vi "Launch PPMS2 UI.vi"() -> ()   [LabVIEW 2016, in "Instrument.PPMS2 UI.lvclass"]
doc: "This will launch a stan-alone user interface for the PPMS 2 Instrument\n\nJKI State Machine Objects (SMO) 1.0.0.5\nJKI - JKI\nCopyright (c) 2016, JKI"
uses:
  Instrument.PPMS2 UI.lvclass
  C:/Program Files (x86)/National Instruments/LabVIEW 2016/vi.lib/JKI/JKI SMO/SMO/SMO.lvclass
  C:/Program Files (x86)/National Instruments/LabVIEW 2016/vi.lib/JKI/JKI SMO/SMO.UI/SMO.UI.lvclass
  instrument.PPMS2/instrument.PPMS2.lvclass
  C:/Program Files (x86)/National Instruments/LabVIEW 2016/user.lib/LevyLab/Levylab Instruments/SMOs/Instrument/Instrument.lvclass
  <vilib>/JKI/JKI SMO/SMO/Typedefs/SMOState --Enum.ctl
  <vilib>/JKI/JKI SMO/SMO/SMO.lvclass
  <vilib>/JKI/JKI SMO/SMO.UI/SMO.UI.lvclass
panel:
  out "error out":errorcluster
  in  "Stop":bool
  # "Launch PPMS 2 UI"
  # "For instructions on how to use the JKI State Machine Objects, examples and video tutorials, visit:\nhttp://jki.net/state-machine-objects/\n\nJKI State Machine Objects™\nhttp://jki.net/state-machine-objects/\nCopyright (C) 2005-2015, JKI <info@jki.net>\nALL RIGHTS RESERVED"
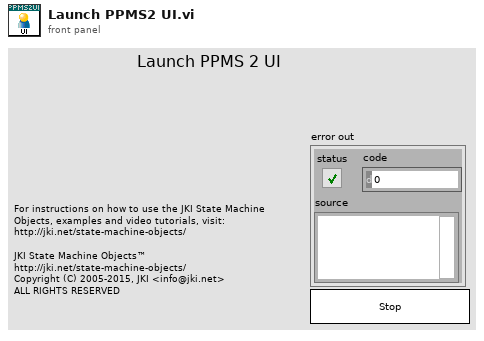
[diagram p1: front panel]
types:
  T1 = typedef "SMO.lvclass/Public Events.ctl" = cluster{"Error":refnum<user-event>, "State":refnum<user-event>, "Reserve State":refnum<user-event>}
  T2 = typedef "SMO.UI.lvclass/PublicEvents--Cluster.ctl" = cluster{"UI Hidden":refnum<user-event>, "UI State":refnum<user-event>}
  T3 = typedef "SMO.lvclass/SMOState --Enum.ctl" = enum16{"unknown", "Created", "Started", "Stopped"}
  T4 = enum32{"Invalid", "Standard", "Closed", "Hidden", "Minimized", "Maximized"}
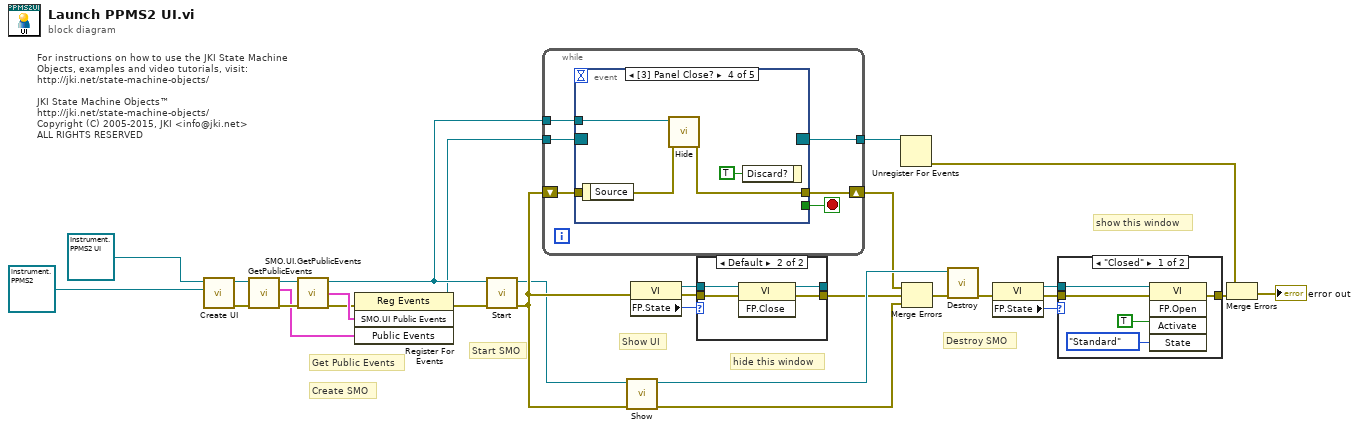
[diagram p0: block diagram]
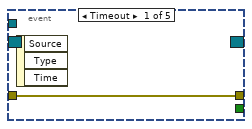
[diagram p4: hidden frame]
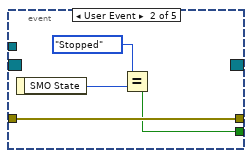
[diagram p5: hidden frame]
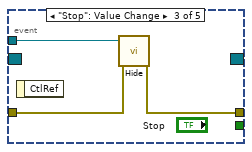
[diagram p6: hidden frame]
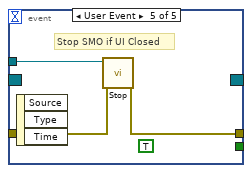
[diagram p7: hidden frame]
diagram:
  # "show this window"
  # "hide this window"
  # "Show UI"
  # "For instructions on how to use the JKI State Machine Objects, examples and video tutorials, visit:\nhttp://jki.net/state-machine-objects/\n\nJKI State Machine Objects™\nhttp://jki.net/state-machine-objects/\nCopyright (C) 2005-2015, JKI <info@jki.net>\nALL RIGHTS RESERVED"
  # "Get Public Events"
  # "Start SMO"
  # "Destroy SMO"
  # "Create SMO"
  n1 = call "Create UI.vi"("Instrument in"=refnum<class "instrument.PPMS2.lvclass"> refnum ("instrument.PPMS2.lvclass"), "Instrument.PPMS2 UI"=refnum<class "Instrument.PPMS2 UI.lvclass"> refnum ("SMO.Template.lvclass")) -> ("error out"=w17:errorcluster, "Instrument.PPMS2 UI out"=w16:refnum<class "Instrument.PPMS2 UI.lvclass">)  [unwired: 8 in]
  n2 = call <vilib>:"GetPublicEvents.vi"("error in (no error)"=w17, "SMO"=w16) -> ("error out"=w19:errorcluster, "Public Events"=w18:T1, "SMO out"=w20:refnum<class "Instrument.PPMS2 UI.lvclass">)  [unwired: 7 in]
  n3 = call <vilib>:"SMO.UI.GetPublicEvents.vi"("error in (no error)"=w19, "SMO.UI"=w20) -> ("error out"=w23:errorcluster, "SMO.UI Public Events"=w24:T2, "SMO.UI out"=w25:refnum<class "Instrument.PPMS2 UI.lvclass">)  [unwired: 7 in]
  n4 = register-events(error in=w23, w24, w18) -> (reference out=w21:refnum<event-registration>, error out=w22:errorcluster)  [unwired: 1 in]
  n5 = call <vilib>:"Start.vi"("error in (no error)"=w22, "SMO"=w25) -> ("error out"=w15:errorcluster, "SMO out"=w3:refnum<class "Instrument.PPMS2 UI.lvclass">)  [unwired: 8 in]
  n6 = while {
    shift-right: [w35] -> w5
    shift-left: w15 -> [w34]
    tunnel: w21 -> [w33]
    tunnel: [w32] -> w30
    tunnel: w25 -> [w31]
    stop <- w36 stop-if-true
    n7 = event shown="[3] Panel Close?" {
      selector: w33 -> [_ _ _ _ _]
      dyn-events: [_ _ _ _ _] -> w32
      timeout: _ -> [_ _ _ _ _]
      tunnel: [_ w38 _ _ _] -> w36
      tunnel: w31 -> [_ _ w44 w47 w51]
      tunnel: [w37 w41 w42 w45 w50] -> w35
      tunnel: w34 -> [w37 w41 w43 w46 w49]
      event Timeout {
        n8 = event-data() -> ()  [unwired: 1 in, 3 out]
      }
      event User Event {
        n9 = event-data() -> ("SMO State"=w40:T3)  [unwired: 1 in]
        n10 = Equal?(x=SMOState_--Enum."Stopped", y=w40) -> (x = y?=w38:bool)
      }
      event "Stop": Value Change {
        n11 = event-data() -> ()  [unwired: 1 in, 1 out]
        n12 = call <vilib>:"Hide.vi"("error in (no error)"=w43, "SMO.UI"=w44) -> ("error out"=w42:errorcluster)  [unwired: 8 in, 1 out]
      }
      event Panel Close? {
        n13 = event-data() -> ()  [unwired: 1 in, 1 out]
        n14 = call <vilib>:"Hide.vi"("error in (no error)"=w46, "SMO.UI"=w47) -> ("error out"=w45:errorcluster)  [unwired: 8 in, 1 out]
        n15 = event-data("Discard?"=TRUE ("OK")) -> ()  [unwired: 1 in, 1 out]
      }
      event User Event {
        (unwired) TRUE ("OK")
        # "Stop SMO if UI Closed"
        n16 = event-data() -> ()  [unwired: 1 in, 3 out]
        n17 = call <vilib>:"Stop.vi"("error in (no error)"=w49, "SMO"=w51) -> ("error out"=w50:errorcluster)  [unwired: 8 in, 1 out]
      }
    }
  }
  n18 = call <vilib>:"Show.vi"("error in (no error)"=w15, "SMO.UI"=w3) -> ("error out"=w4:errorcluster, "SMO.UI out"=w27:refnum<class "Instrument.PPMS2 UI.lvclass">)  [unwired: 8 in]
  n19 = property class="VI"(error in=w15) -> (reference out=w13:refnum<vi>, error out=w14:errorcluster, "FP.State"=w12:T4)  [unwired: 1 in]
  n20 = case shown="Default" w12 {
    tunnel: [w53 w57] -> w6
    tunnel: w14 -> [w53 w56]
    tunnel: w13 -> [w52 w55]
    tunnel: [w52 w54] -> _
    frame "Invalid", "Closed" {
    }
    frame Default {
      n21 = invoke class="VI" method="FP.Close"(reference=w55, error in=w56) -> (reference out=w54:refnum<vi>, error out=w57:errorcluster)  [unwired: 1 in, 1 out]
    }
  }
  n22 = Unregister For Events(event registration refnum=w30) -> (error out=w29:errorcluster)  [unwired: 1 in]
  n23 = Merge Errors(w5, w6, w4) -> (w26:errorcluster)
  n24 = call <vilib>:"Destroy.vi"("error in (no error)"=w26, "SMO"=w27) -> ("error out"=w8:errorcluster)  [unwired: 9 in]
  n25 = property class="VI"(error in=w8) -> (reference out=w9:refnum<vi>, error out=w10:errorcluster, "FP.State"=w11:T4)  [unwired: 1 in]
  n26 = case shown="\"Closed\"" w11 {
    tunnel: [w60 w63] -> w7
    tunnel: w10 -> [w59 w63]
    tunnel: w9 -> [w58 _]
    frame "Closed" {
      n27 = invoke class="VI" method="FP.Open"(reference=w58, error in=w59, "Activate"=TRUE, "State"=T4."Standard") -> (error out=w60:errorcluster)  [unwired: 1 in, 4 out]
    }
    frame Default {
    }
  }
  n28 = Merge Errors(w29, w7) -> (→"error out":errorcluster)
